vi "Read Sub Export Build Order.vi"(8 "error in (no error)":errorcluster, 11 "Compound_Installer in":refnum<class "Compound_Installer.lvclass">) -> (0 "error out":errorcluster, 2 "Sub Export Build Order":string[](array[string]), 3 "Compound_Installer out":refnum<class "Compound_Installer.lvclass">)   [LabVIEW 2017, in "CL_G3_VIComponentBuilder.lvlib" / "Compound_Installer.lvclass"]
uses:
  Compound_Installer.lvclass
  Compound_Installer.lvclass/Compound_Installer.ctl
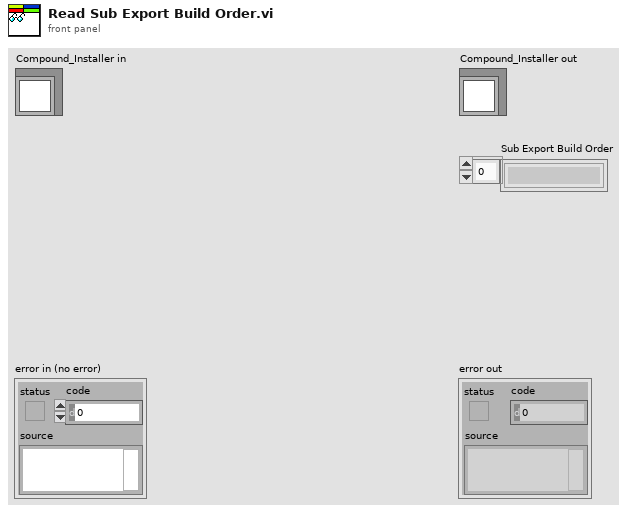
[diagram p1: front panel]
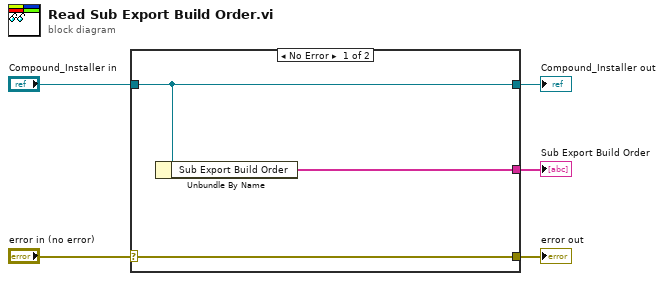
[diagram p0: block diagram]
diagram:
  n1 = case shown="No Error" "error in (no error)" {
    selector: "error in (no error)" -> [w8 w9]
    tunnel: [w8 w9] -> w4
    tunnel: [w7 w10] -> w2
    tunnel: "Compound_Installer in" -> [w7 w10]
    tunnel: [w6 _] -> w1
    frame No Error {
      n2 = Unbundle By Name(w7) -> ("Sub Export Build Order"=w6:string[])
    }
    frame Error {
    }
  }
  "error out" <- w4
  "Compound_Installer out" <- w2
  "Sub Export Build Order" <- w1
